vi "Command (write) - SP.vi"(7 "timeout ms (100)":i32=100, 8 "error in (no error)":errorcluster, 9 "Position":i32, 10 "IP":string, 11 "connection ID in":refnum<k16>) -> (0 "error out":errorcluster, 3 "connection ID out":refnum<k16>)   [LabVIEW 2016, in "SMD-7615.lvlib" / "eSCL.lvlib"]
doc: "SP - Set Position\nSets or requests the motor’s absolute position. To ensure that the internal position counter resets properly, use EP immediately prior to sending SP. For example, to set the position to zero after a homing routine, send EP0 immediately followed by SP0."
uses:
  eSCL.lvlib
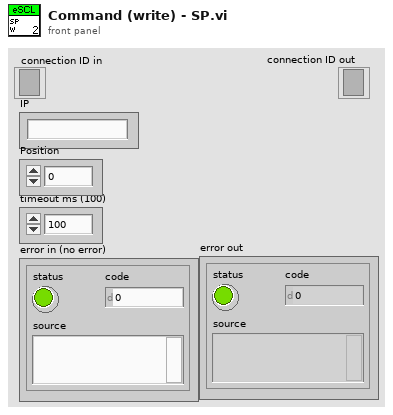
[diagram p1: front panel]
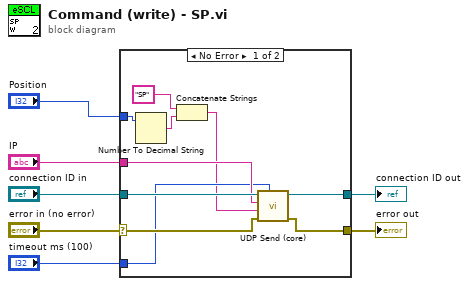
[diagram p0: block diagram]
diagram:
  n1 = case shown="No Error" "error in (no error)" {
    selector: "error in (no error)" -> [w17 w18]
    tunnel: "connection ID in" -> [w16 w19]
    tunnel: [w12 w19] -> w5
    tunnel: [w11 w18] -> w4
    tunnel: "IP" -> [w15 _]
    tunnel: "timeout ms (100)" -> [w14 _]
    tunnel: "Position" -> [w9 _]
    frame No Error {
      n2 = Number To Decimal String(number=w9) -> (decimal integer string=w8:string)  [unwired: 1 in]
      n3 = Concatenate Strings("SP" ("Data"), w8) -> (w10:string)
      n4 = call "UDP Send (core).vi"("timeout ms (100)"=w14, "error in (no error)"=w17, "Data"=w10, "IP"=w15, "connection ID in"=w16) -> ("error out"=w11:errorcluster, "connection ID out"=w12:refnum<k16>)  [unwired: 5 in]
    }
    frame Error {
    }
  }
  "connection ID out" <- w5
  "error out" <- w4
